vi "PM_Sync2Tekron.vi"(0 "instrument handle in":refnum<k15>, 3 "error in":errorcluster) -> (7 "instrument handle out":refnum<k15>, 8 "802.1AS Monitor":string[][](table), 9 "Synchronized":bool, 10 "error out":errorcluster)   [LabVIEW 2021]
panel:
  out "References Type":string[](array[string])
  in  "BMCA Mode":i32(ring) items=["SlaveOnly", "MasterSlave"]
  in  "1588:Clock Accuracy":i32(ring) items=["Unknown", "Within25nsec", "Within100nsec", "Within250nsec", "Within1usec", "Within2500nsec", "Within10usec", "Within25usec", "Within100usec", "Within250usec", "Within1msec", "Within2500usec", "Within10msec", "Within25msec", "Within100msec", "Within250msec", "Within1sec", "Within10sec", "GreaterThan10sec"]
  in  "Clock State":i32(ring) items=["Initializing", "Faulty", "Disabled", "Listening", "PreMaster", "Master", "Passive", "Uncalibrated", "Slave", "Stopped"]
  out "Grandmaster Clock ID":string
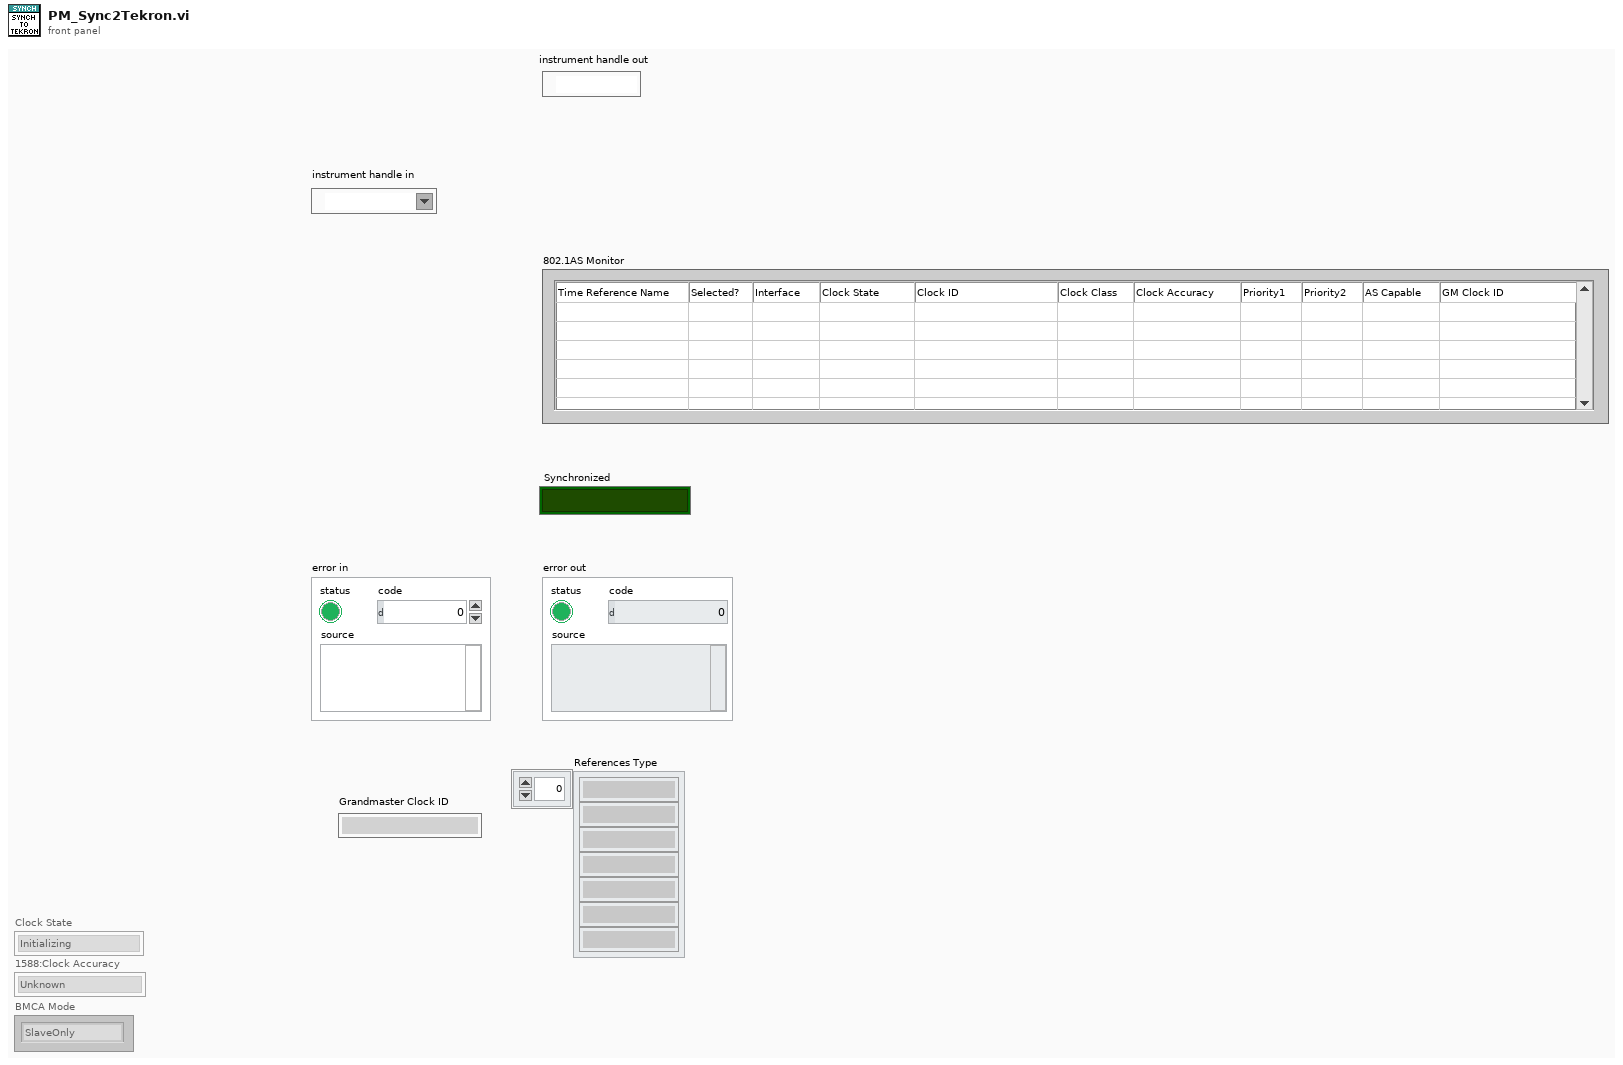
[diagram p1: front panel]
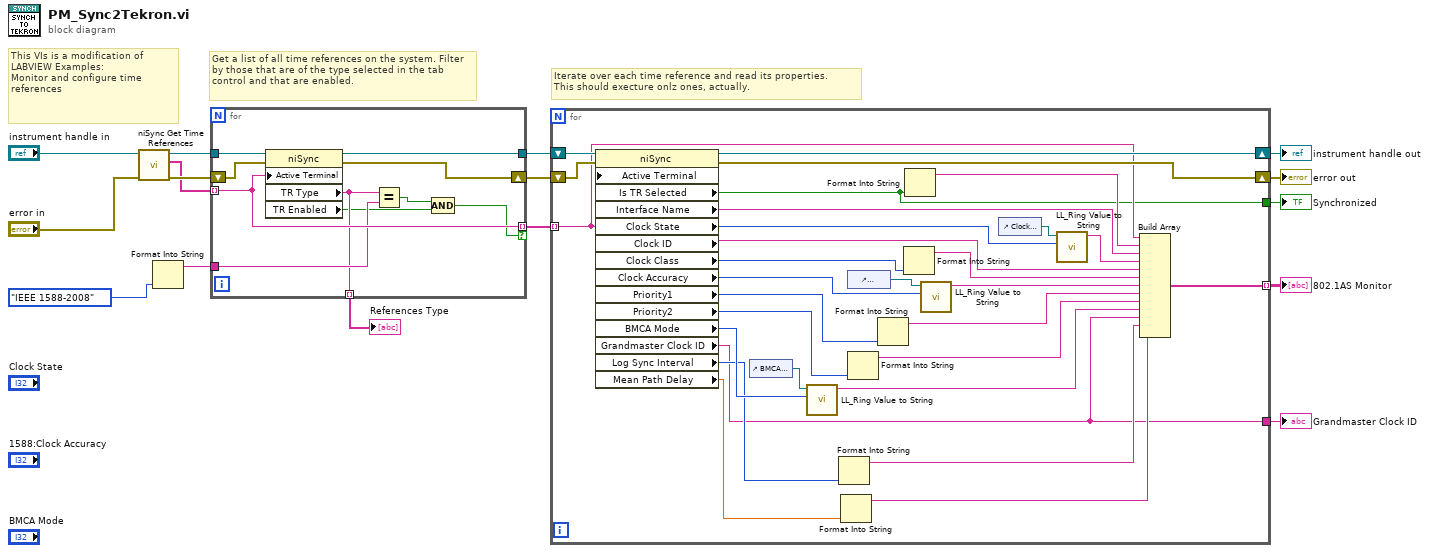
[diagram p0: block diagram]
diagram:
  # "This VIs is a modification of LABVIEW Examples: \nMonitor and configure time references"
  # "Iterate over each time reference and read its properties.\nThis should execture onlz ones, actually."
  # "Get a list of all time references on the system. Filter by those that are of the type selected in the tab control and that are enabled."
  n1 = call <instrlib>:"niSync Get Time References.vi"("error in (no error)"="error in", "instrument handle"="instrument handle in") -> ("error out"=w15:errorcluster, "time references"=w14:string[], "instrument handle out"=w16:refnum<k15>)  [unwired: 7 in]
  n2 = Format Into String(enum32{"IEEE 1588-2008", "IEEE 802.1AS-2011"}."IEEE 1588-2008" ("input 1")) -> (resulting string=w12:string)  [unwired: 3 in, 1 out]
  n3 = for {
    tunnel: w16 -> [w26]
    tunnel: w14 -> [w24] mode=indexing
    tunnel: w12 -> [w21]
    tunnel: [w24] -> w1 mode=indexing if=w17
    tunnel: [w23] -> w8
    shift-right: [w22] -> w13
    shift-left: w15 -> [w25]
    tunnel: [w20] -> w2 mode=indexing
    n4 = property class="niSync"(reference=w26, error in=w25, "Active Terminal"=w24) -> (reference out=w23:refnum<k15>, error out=w22:errorcluster, "TR Type"=w20:string, "TR Enabled"=w18:bool)
    n5 = Equal?(x=w20, y=w21) -> (x = y?=w19:bool)
    n6 = Compound Arithmetic op=AND(w19, w18) -> (w17:bool)
  }
  "References Type" <- w2
  n7 = for {
    tunnel: w1 -> [w34] mode=indexing
    shift-right: [w37] -> w9
    shift-left: w13 -> [w54]
    tunnel: [w53] -> w3 mode=indexing
    shift-right: [w55] -> w4
    shift-left: w8 -> [w56]
    tunnel: [w28] -> w10
    tunnel: [w27] -> w11
    n8 = property class="niSync"(reference=w56, error in=w54, "Active Terminal"=w34) -> (reference out=w55:refnum<k15>, error out=w37:errorcluster, "Is TR Selected"=w27:bool, "Interface Name"=w36:string, "Clock State"=w49:i32, "Clock ID"=w47:string, "Clock Class"=w52:i32, "Clock Accuracy"=w51:i32, "Priority1"=w50:i32, "Priority2"=w41:i32, "BMCA Mode"=w40:i32, "Grandmaster Clock ID"=w28:string, "Log Sync Interval"=w32:i32, "Mean Path Delay"=w30:dbl)
    n9 = control-ref of="BMCA Mode"() -> (w33:refnum<vi>)
    n10 = call "LL_Ring Value to String.vi"("Value"=w40, "Ring in"=w33) -> ("String"=w39:string)  [unwired: 9 in]
    n11 = Format Into String(w32) -> (resulting string=w31:string)  [unwired: 3 in, 1 out]
    n12 = Format Into String(w30) -> (resulting string=w29:string)  [unwired: 3 in, 1 out]
    n13 = control-ref of="1588:Clock Accuracy"() -> (w42:refnum<vi>)
    n14 = Format Into String(w41) -> (resulting string=w43:string)  [unwired: 3 in, 1 out]
    n15 = Format Into String(w50) -> (resulting string=w44:string)  [unwired: 3 in, 1 out]
    n16 = Format Into String(w52) -> (resulting string=w46:string)  [unwired: 3 in, 1 out]
    n17 = Format Into String(w27) -> (resulting string=w35:string)  [unwired: 3 in, 1 out]
    n18 = call "LL_Ring Value to String.vi"("Value"=w51, "Ring in"=w42) -> ("String"=w45:string)  [unwired: 9 in]
    n19 = control-ref of="Clock State"() -> (w38:refnum<vi>)
    n20 = call "LL_Ring Value to String.vi"("Value"=w49, "Ring in"=w38) -> ("String"=w48:string)  [unwired: 9 in]
    n21 = Build Array(w34, w35, w36, w48, w47, w46, w45, w44, w43, w39, w28, w31, w29) -> (w53:string[])
  }
  "Grandmaster Clock ID" <- w10
  "Synchronized" <- w11
  "instrument handle out" <- w4
  "error out" <- w9
  "802.1AS Monitor" <- w3
